vi "Interpret Deviation Signal From Raw Data.vi"   [LabVIEW 2013]
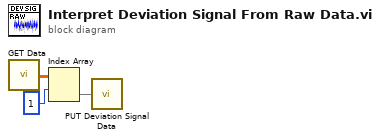
[diagram p0: block diagram]
diagram:
  n1 = call "GET Data.vi"() -> ("Data"=w3:dbl[][])
  n2 = Index Array(array=w3, index (row)=1) -> (element=w1:dbl[])  [unwired: 1 in]
  n3 = call "PUT Deviation Signal Data.vi"("Deviation Signal Data"=w1) -> ()
